vi "Grip System.vi"   [LabVIEW 2018]
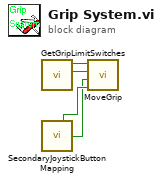
[diagram p0: block diagram]
diagram:
  n1 = call "GetGripLimitSwitches.vi"() -> ("Close Limit Switch"=w3:bool, "Open Limit Switch"=w4:bool)  [unwired: 10 in]
  n2 = call "SecondaryJoystickButtonMapping.vi"() -> ("Close Grip"=w2:bool, "Open Grip"=w1:bool)  [unwired: 9 in, 5 out]
  n3 = call "MoveGrip.vi"("Close Button"=w2, "Open Button"=w1, "Close Limit Switch"=w3, "Open Limit Switch"=w4) -> ()  [unwired: 8 in]
